vi "Config.INI, Read_Write, Path.vi"(5 "Read(F)/Write(T)":bool, 7 "Section":string, 8 "error in":errorcluster, 9 "Value/DefaultValue":path, 10 "Key":string="DefaultDataFolder", 11 "refnum":T1) -> (0 "error out":errorcluster, 1 "Value Out":path, 2 "found?":bool, 3 "refnum out":T1)   [LabVIEW 2018]
uses:
  <vilib>/Utility/config.llb/Config Data RefNum.ctl
  <vilib>/Utility/config.llb/Read Key (Path).vi
  <vilib>/Utility/config.llb/Write Key (Path).vi
  <vilib>/Utility/config.llb/NI_LVConfig.lvlib
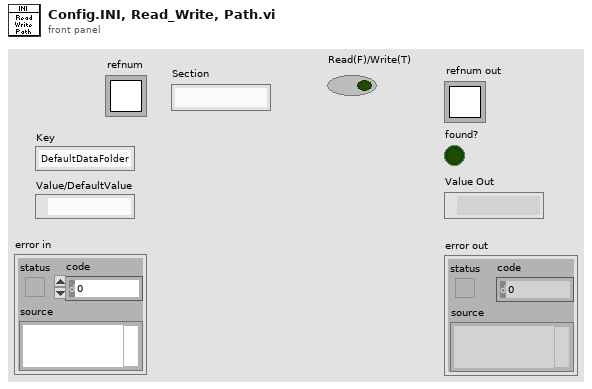
[diagram p1: front panel]
types:
  T1 = typedef "NI_LVConfig.lvlib/Config Data RefNum.ctl" = refnum<k1>
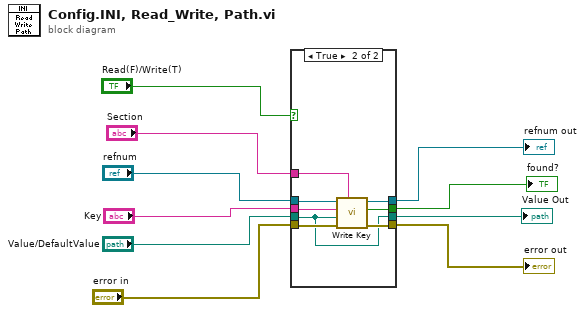
[diagram p0: block diagram]
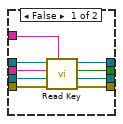
[diagram p2: hidden frame]
diagram:
  n1 = case shown="True" "Read(F)/Write(T)" {
    tunnel: "Key" -> [w19 w23]
    tunnel: "Value/DefaultValue" -> [w18 w20]
    tunnel: [w17 w20] -> w8
    tunnel: "refnum" -> [w16 w26]
    tunnel: "Section" -> [w15 w24]
    tunnel: [w14 w25] -> w5
    tunnel: [w13 w21] -> w4
    tunnel: [w12 w27] -> w3
    tunnel: "error in" -> [w11 w22]
    frame False {
      n2 = call-poly <vilib>:"Read Key.vi"("section"=w15, "error in (no error)"=w11, "default value"=w18, "key"=w19, "refnum"=w16) -> ("error out"=w12:errorcluster, "value"=w17:path, "found?"=w13:bool, "refnum out"=w14:T1)  [unwired: 3 in]
    }
    frame True {
      n3 = call-poly <vilib>:"Write Key.vi"("section"=w24, "error in (no error)"=w22, "value"=w20, "key"=w23, "refnum"=w26) -> ("error out"=w27:errorcluster, "found?"=w21:bool, "refnum out"=w25:T1)  [unwired: 4 in]
    }
  }
  "Value Out" <- w8
  "refnum out" <- w5
  "found?" <- w4
  "error out" <- w3
